vi "PH_Tektronix_7000.get Trigger Configuration.vi"(0 "i ref in":refnum<vi>, 5 "error IO":errorcluster) -> (14 "i ref out":refnum<vi>, 19 "error out":errorcluster)   [LabVIEW 2014, in "PH_Tektronix_7000.lvlib"]
doc: "If the connection is established, the trigger configuration is set and written to own attributes as well as the errors."
uses:
  PH_Tektronix_7000.lvlib
  PH_Tektronix_7000.Trigger Config.ctl
  instr.lib/Tektronix7000Series/Tektronix 7000 Series - Driver np.lvlib
panel:
  in  "Trigger Configuration":T1 {"Trigger Mode" items=["Normal", "Auto"]; "Coupling" items=["DC", "AC", "Hf Reject", "Lf Reject", "Noise Rej", "Atrigger"]; "Slope" items=["Rise", "Fall", "Either"]; "Source" items=["Channel1"=0, "Channel2"=1, "Channel3"=2, "Channel4"=3, "Aux"=12, "Line"=13]}
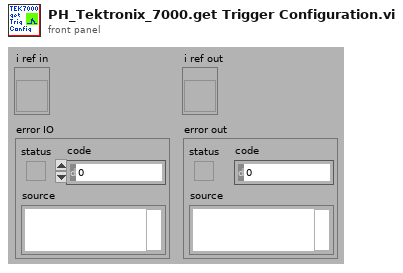
[diagram p1: front panel]
types:
  T1 = typedef "PH_Tektronix_7000.lvlib/PH_Tektronix_7000.Trigger Config.ctl" = cluster{"Source":u16, "Level [V]":dbl, "Slope":u16, "Coupling":u16, "Trigger Mode":u16}
  T2 = typedef "PH_Tektronix_7000.lvlib/PH_Tektronix_7000.i attribute.ctl" = cluster{"VISA Resource Name":refnum<visa-resource-name>, "IDN":cluster{"Instrument Driver":string, "Instrument Firmware":string, "Model":string, "Serial Number":string}, "Selftest":cluster{"Result":i32, "Message":string}, "Trigger Configuration":T1, "Acquisition Configuration":T3, "GUI Refs":T4, "State":T5, "Error Message":string, "Allow Prdc Loop?":bool, "Channel 1":T6, "Channel 2":T6, "Channel 3":T6, "Channel 4":T6, "Data CH 1":waveform(dbl), "Data CH 2":waveform(dbl), "Data CH 3":waveform(dbl), "Data CH 4":waveform(dbl), "Allow config?":bool, "Name Channel 1":string, "Name Channel 2":string, "Name Channel 3":string, "Name Channel 4":string, "Fetch Data before sending to PSDB?":bool, "Constructor passed?":bool, "Data taken at":timestamp, "Plot Colors":u32[], "Default VISA Resource":string}
  T3 = typedef "PH_Tektronix_7000.lvlib/PH_Tektronix_7000.Acquisition Config.ctl" = cluster{"Record Length":u32, "Timebase [s/div]":dbl, "Position [%]":dbl, "Acquisition Type":u16, "Average Waveforms":i32, "Envelope Waveforms":i32, "WfmDB Samples":i32, "Continuous?":bool, "Delay [s]":dbl, "Run?":bool}
  T4 = typedef "PH_Tektronix_7000.lvlib/PH_Tektronix_7000.GUI Refs.ctl" = cluster{"Graph":refnum<vi>, "State":refnum<vi>, "Delete":refnum<vi>, "VISA Resource":refnum<vi>, "Allow Configure":refnum<vi>, "Fetch Data":refnum<vi>, "Fetch before sending Data to PSDB":refnum<vi>, "Name Channel 1":refnum<vi>, "Name Channel 2":refnum<vi>, "Name Channel 3":refnum<vi>, "Name Channel 4":refnum<vi>, "Prdc Intervall [ms]":refnum<vi>, "Data taken":refnum<vi>, "Model":refnum<vi>, "Serial Number":refnum<vi>, "Firmware":refnum<vi>, "Driver":refnum<vi>, "Acquisition":refnum<vi>, "Trigger":refnum<vi>, "Cursor: D Time [s]":refnum<vi>, "Cursor: D Signal [V]":refnum<vi>, "Channel 1":refnum<vi>, "Channel 2":refnum<vi>, "Channel 3":refnum<vi>, "Channel 4":refnum<vi>}
  T5 = typedef "PH_StatusHandler.lvlib/PH_StatusHandler.Status.ctl" = i16
  T6 = typedef "PH_Tektronix_7000.lvlib/PH_Tektronix_7000.Channel Config.ctl" = cluster{"Enable Channel":bool, "Bandwidth":u16, "Input Impedance":u16, "Vertical Coupling":u16, "Probe Attenuation":dbl, "Range [V/div]":dbl, "Position [div]":dbl, "Bandwidth raw":string}
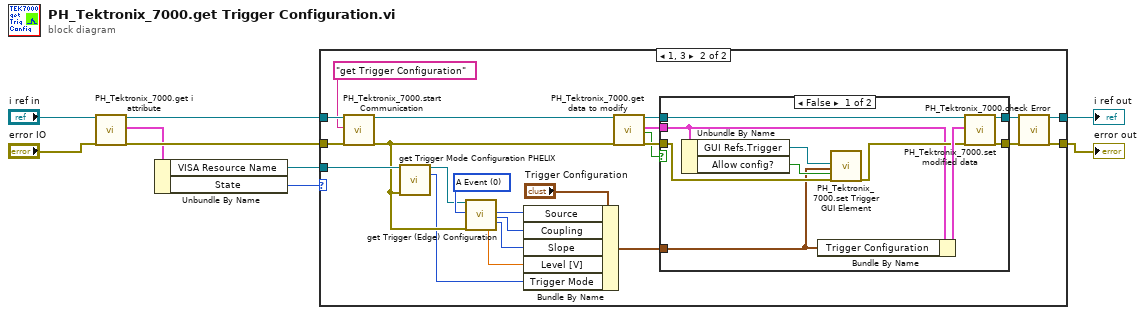
[diagram p0: block diagram]
diagram:
  n1 = call "PH_Tektronix_7000.get i attribute.vi"("i ref in"="i ref in", "error in (no error)"="error IO") -> ("i ref out"=w4:refnum<vi>, "i attribute"=w6:T2, "error out"=w8:errorcluster)  [unwired: 15 in]
  n2 = Unbundle By Name(w6) -> ("VISA Resource Name"=w7:refnum<visa-resource-name>, "State"=w1:T5)
  n3 = case shown="1, 3" w1 {
    tunnel: w4 -> [w11 w28]
    tunnel: w7 -> [_ w22]
    tunnel: [w10 w26] -> w2
    tunnel: w8 -> [w10 w29]
    tunnel: [w11 w24] -> w9
    frame Default {
    }
    frame 1, 3 {
      w15 = u16 0 items=["A Event", "B Event"] ("Trigger Event (0:A Event)")
      n4 = call "PH_Tektronix_7000.start Communication.vi"("i ref in"=w28, "Action"="get Trigger Configuration", "error in"=w29) -> ("i ref out"=w27:refnum<vi>, "error out"=w13:errorcluster)  [unwired: 15 in]
      n5 = call "get Trigger Mode Configuration PHELIX.vi"("VISA resource name"=w22, "error in (no error)"=w13) -> ("VISA resource name out"=w14:refnum<visa-resource-name>, "Trigger Mode"=w12:u16)  [unwired: 11 in, 1 out]
      n6 = call "get Trigger (Edge) Configuration.vi"("VISA resource name"=w14, "Trigger Event (0:A Event)"=w15, "error in (no error)"=w13) -> ("Trigger Level[V]"=w17:dbl, "Trigger Source"=w20:u16, "Trigger Coupling"=w19:u16, "Trigger Slope"=w18:u16)  [unwired: 7 in, 6 out]
      n7 = Bundle By Name(cluster="Trigger Configuration", "Source"=w20, "Coupling"=w19, "Slope"=w18, "Level [V]"=w17, "Trigger Mode"=w12) -> (w16:T1)
      n8 = call "PH_Tektronix_7000.get data to modify.vi"("i ref in"=w27, "error in (no error)"=w13) -> ("i ref out"=w32:refnum<vi>, "i attribute"=w30:T2, "timed out"=w31:bool, "error out"=w33:errorcluster)  [unwired: 14 in]
      n9 = case shown="False" w31 {
        tunnel: [w44 w45] -> w34
        tunnel: w33 -> [w43 w45]
        tunnel: w32 -> [w42 w46]
        tunnel: [w41 w46] -> w25
        tunnel: w30 -> [w38 _]
        tunnel: w16 -> [w35 _]
        frame False {
          n10 = Unbundle By Name(w38) -> ("GUI Refs.Trigger"=w36:refnum<vi>, "Allow config?"=w37:bool)
          n11 = Bundle By Name(cluster=w38, "Trigger Configuration"=w35) -> (w40:T2)
          n12 = call "PH_Tektronix_7000.set Trigger GUI Element.vi"("Ref Trigger Config"=w36, "Trigger Config"=w35, "Enabled?"=w37, "error in"=w43) -> ("error out"=w39:errorcluster)  [unwired: 15 in]
          n13 = call "PH_Tektronix_7000.set modified data.vi"("i ref in"=w42, "i attribute"=w40, "error in (no error)"=w39) -> ("i ref out"=w41:refnum<vi>, "error out"=w44:errorcluster)  [unwired: 15 in]
        }
        frame True {
        }
      }
      n14 = call "PH_Tektronix_7000.check Error.vi"("i ref in"=w25, "error in"=w34) -> ("i ref out"=w24:refnum<vi>, "error out"=w26:errorcluster)  [unwired: 16 in]
    }
  }
  "i ref out" <- w9
  "error out" <- w2
